vi "ICR_Initialize_Panel.vi"(8 "error in (no error)":errorcluster caption="entrée d'erreur (pas d'erreur)", 11 "QMH ICR Cluster":T1) -> (0 "error out":errorcluster caption="sortie d'erreur", 3 "QMH ICR Cluster":T1)   [LabVIEW 2020]
uses:
  controls/QMH_ICR_Cluster.ctl
  controls/HARDWARE_Resources.ctl
  controls/PROCESSING_Inputs.ctl
  controls/LOOPS_Inputs.ctl
  controls/OPO_Inputs.ctl
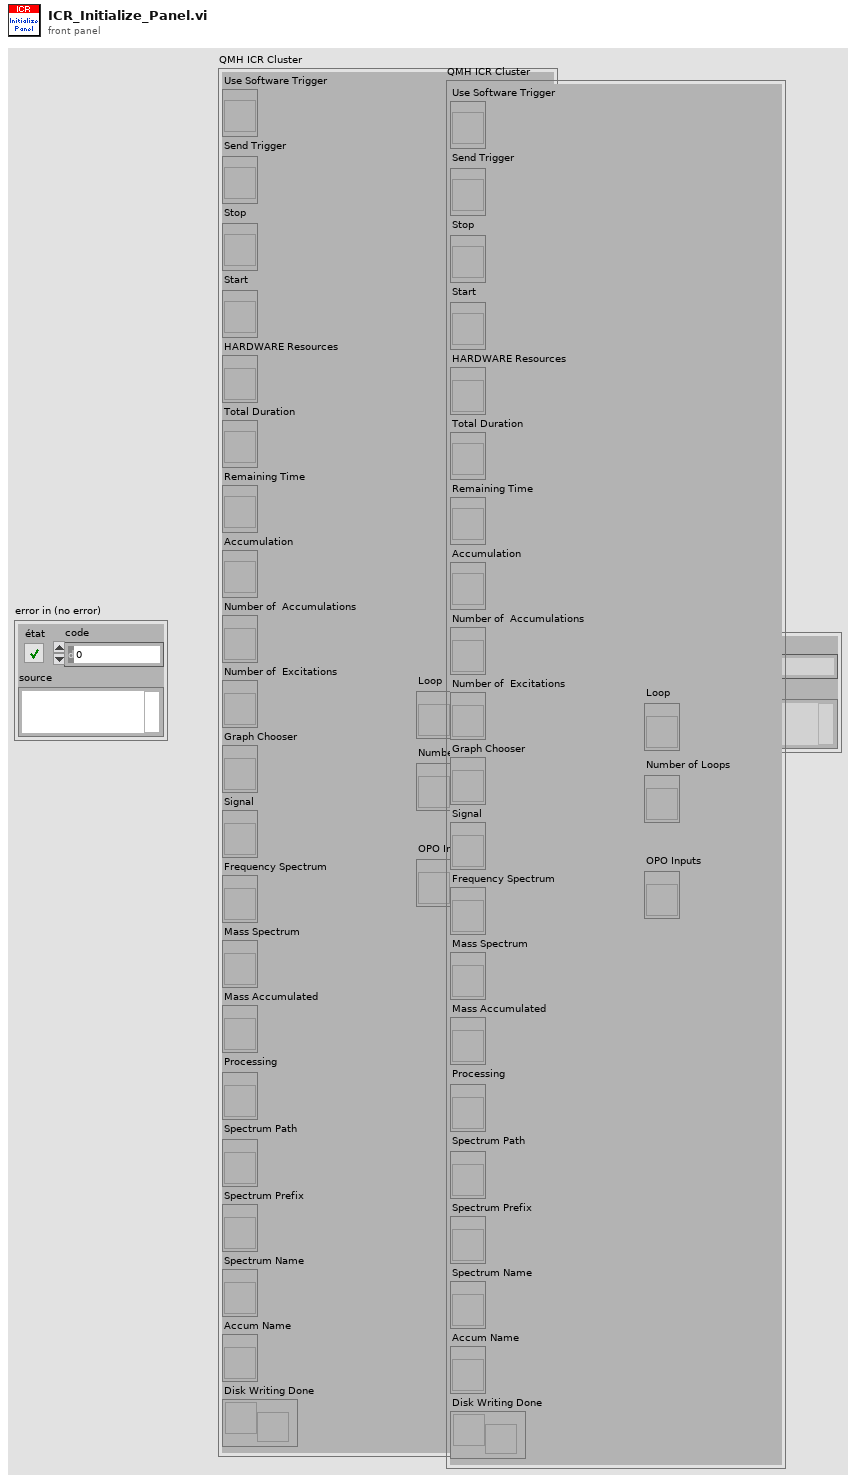
[diagram p1: front panel]
types:
  T1 = typedef "QMH_ICR_Cluster.ctl" = cluster{"Use Software Trigger":refnum<vi>, "Send Trigger":refnum<vi>, "Stop":refnum<vi>, "Start":refnum<vi>, "HARDWARE Resources":refnum<vi>, "Total Duration":refnum<vi>, "Remaining Time":refnum<vi>, "Accumulation":refnum<vi>, "Number of  Accumulations":refnum<vi>, "Number of  Excitations":refnum<vi>, "Graph Chooser":refnum<vi>, "Signal":refnum<vi>, "Frequency Spectrum":refnum<vi>, "Mass Spectrum":refnum<vi>, "Mass Accumulated":refnum<vi>, "Processing":refnum<vi>, "Spectrum Path":refnum<vi>, "Spectrum Prefix":refnum<vi>, "Spectrum Name":refnum<vi>, "Accum Name":refnum<vi>, "Disk Writing Done":refnum<notifier>, "Loop":refnum<vi>, "Number of Loops":refnum<vi>, "OPO Inputs":refnum<vi>}
  T2 = enum32{"Signal", "Frequency Spectrum", "Mass Spectrum"}
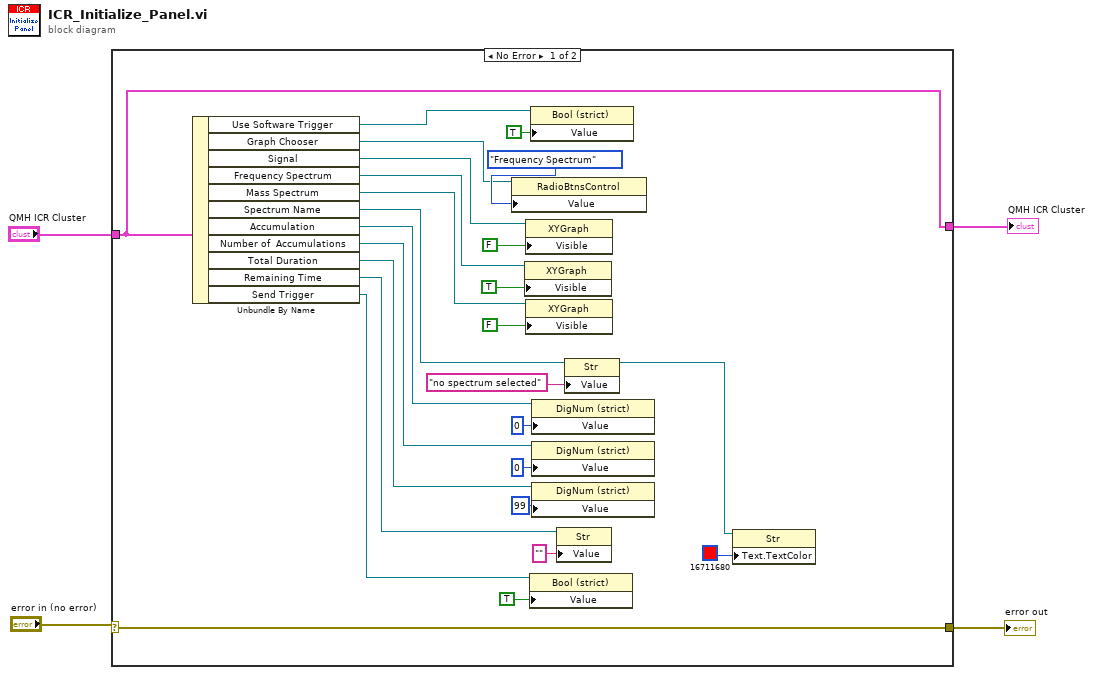
[diagram p0: block diagram]
diagram:
  n1 = case shown="No Error" "error in (no error)" {
    selector: "error in (no error)" -> [w30 w32]
    tunnel: "QMH ICR Cluster" -> [w9 w31]
    tunnel: [w30 w32] -> w3
    tunnel: [w9 w31] -> w1
    frame No Error {
      n2 = Unbundle By Name(w9) -> ("Use Software Trigger"=w19:refnum<vi>, "Graph Chooser"=w20:refnum<vi>, "Signal"=w21:refnum<vi>, "Frequency Spectrum"=w22:refnum<vi>, "Mass Spectrum"=w23:refnum<vi>, "Spectrum Name"=w24:refnum<vi>, "Accumulation"=w17:refnum<vi>, "Number of  Accumulations"=w14:refnum<vi>, "Total Duration"=w13:refnum<vi>, "Remaining Time"=w11:refnum<vi>, "Send Trigger"=w6:refnum<vi>)
      n3 = property class="RadioBtnsControl"(reference=w20, "Value"=T2."Frequency Spectrum" ("Valeur")) -> ()  [unwired: 1 in, 2 out]
      n4 = property class="XYGraph"(reference=w22, "Visible"=TRUE) -> ()  [unwired: 1 in, 2 out]
      n5 = property class="XYGraph"(reference=w21, "Visible"=FALSE) -> ()  [unwired: 1 in, 2 out]
      n6 = property class="XYGraph"(reference=w23, "Visible"=FALSE) -> ()  [unwired: 1 in, 2 out]
      n7 = property class="Bool (strict)"(reference=w6, "Value"=TRUE) -> ()  [unwired: 1 in, 2 out]
      n8 = property class="Bool (strict)"(reference=w19, "Value"=TRUE ("Valeur")) -> ()  [unwired: 1 in, 2 out]
      n9 = property class="DigNum (strict)"(reference=w17, "Value"=0 ("Valeur")) -> ()  [unwired: 1 in, 2 out]
      n10 = property class="DigNum (strict)"(reference=w14, "Value"=0 ("Valeur")) -> ()  [unwired: 1 in, 2 out]
      n11 = property class="DigNum (strict)"(reference=w13, "Value"=99) -> ()  [unwired: 1 in, 2 out]
      n12 = property class="Str"(reference=w11, "Value"="" ("Valeur")) -> ()  [unwired: 1 in, 2 out]
      n13 = property class="Str"(reference=w24, "Value"="no spectrum selected" ("Valeur")) -> (reference out=w7:refnum<vi>)  [unwired: 1 in, 1 out]
      n14 = property on="Nœud de propriété" class="Str"(reference=w7, "Text.TextColor"=u32 16711680) -> ()  [unwired: 1 in, 2 out]
    }
    frame Error {
    }
  }
  "error out" <- w3
  "QMH ICR Cluster" <- w1
